vi "Set Serial Break Event.vi"() -> ()   [LabVIEW 2023]
doc: "This example illustrates how to introduce a break in the data line during serial communication. The VISA Serial Break VI is used to introduce a break in the data line. This VI can be run alongside the Detect Serial Break Event example on a separate serial port to monitor the breaks.\n\nThe serial break is a condition that holds the transmit line logic-low for longer than one data byte. Normally, if there's no data to transmit, then the transmit line idle condition is logic-high. Your application may require that you send a serial break in the transmission line. You can use this example to provide that capability to a particular device. Alternatively, you can use this example to test the Detect Serial Break Event example."
uses:
  support/Serial - Settings.ctl
  <vilib>/Instr/_visa.llb/VISA Configure Serial Port (Instr).vi
  <vilib>/Instr/_visa.llb/VISA Serial Break (Instr).vi
panel:
  in  "Serial Settings":T1={"baud rate"=9600, "data bits"=8, "parity"=enum."None", "stop bits"=10, "flow control"=0} {"flow control" items=["None"=0, "XON/XOFF"=1, "RTS/CTS"=2, "DTR/DSR"=4]; "stop bits" items=["1.0"=10, "1.5"=15, "2.0"=20]; "data bits" min=5 max=8 step=1; "baud rate" items=["75"=75, "110"=110, "134"=134, "150"=150, "300"=300, "600"=600, "1200"=1200, "1800"=1800, "2400"=2400, "4800"=4800, "7200"=7200, "9600"=9600, "14400"=14400, "19200"=19200, "28800"=28800, "38400"=38400, "56000"=56000, "57600"=57600, "115200"=115200, "128000"=128000, "230400"=230400]}
  in  "break length":i16=250 min=1 max=500
  in  "Set Break":bool
  in  "Stop":bool
  in  "VISA resource name":refnum<visa-resource-name>="COM1"
  # "Overview: Demonstrates the use of the VISA functions to set a break in the line during serial communication.\nRequirements: NI-VISA Driver, multiple serial ports\nInstructions:\n1. Ensure Detect Serial Break Event.vi is already running.\n2. Ensure that the VISA resource name values in both VIs are set to different serial ports that are connected to each other.\n3. Run the VI.\n4. Click the Set Break button and observe the front panel of Detect Serial Break Event.vi. You should see the Break Detected? light come on, and the Number of Breaks indicator increment by 1.\n5. Click Stop to stop the VI."
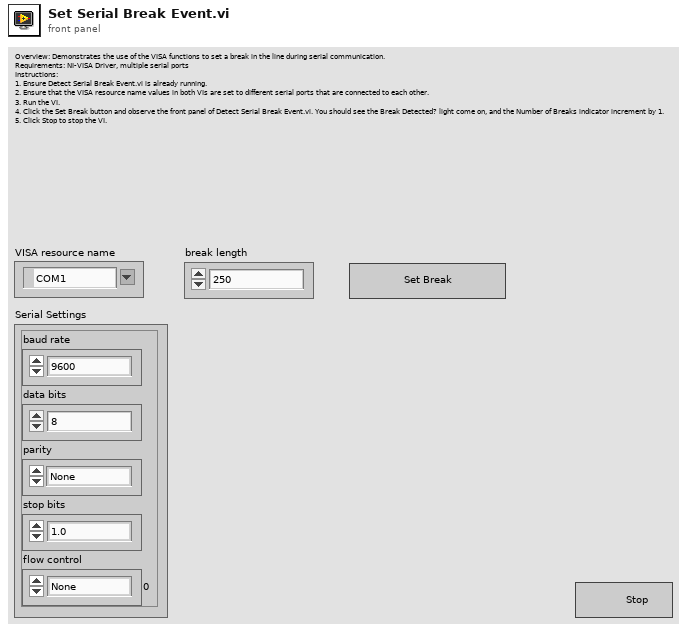
[diagram p1: front panel]
types:
  T1 = typedef "Serial - Settings.ctl" = cluster{"baud rate":u32, "data bits":u16, "parity":enum16{"None", "Odd", "Even", "Mark", "Space"}, "stop bits":u16, "flow control":u16}
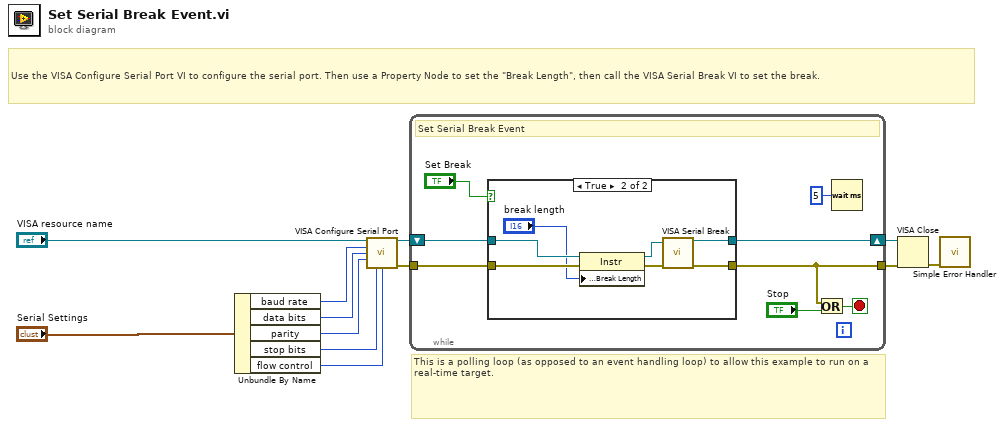
[diagram p0: block diagram]
diagram:
  # "This is a polling loop (as opposed to an event handling loop) to allow this example to run on a real-time target."
  # "Use the VISA Configure Serial Port VI to configure the serial port. Then use a Property Node to set the \"Break Length\", then call the VISA Serial Break VI to set the break."
  n1 = Unbundle By Name("Serial Settings") -> ("baud rate"=w5:u32, "data bits"=w4:u16, "parity"=w3:enum16{"None", "Odd", "Even", "Mark", "Space"}, "stop bits"=w2:u16, "flow control"=w1:u16)
  n2 = call-poly "VISA Configure Serial Port"("VISA resource name"="VISA resource name", "baud rate (9600)"=w5, "data bits (8)"=w4, "parity (0:none)"=w3, "stop bits (10: 1 bit)"=w2, "flow control (0:none)"=w1) -> ("VISA resource name out"=w11:refnum<visa-resource-name>, "error out"=w10:errorcluster)  [unwired: 3 in, 5 out]
  n3 = while {
    tunnel: w10 -> [w19]
    tunnel: [w17] -> w9
    shift-right: [w18] -> w8
    shift-left: w11 -> [w20]
    stop <- w16 stop-if-true
    # "Set Serial Break Event"
    n4 = case shown="True" "Set Break" {
      tunnel: w20 -> [w21 w29]
      tunnel: w19 -> [w22 w28]
      tunnel: [w21 w27] -> w18
      tunnel: [w22 w26] -> w17
      frame False {
      }
      frame True {
        n5 = property class="Instr"(reference=w29, error in=w28, "Serial Settings:Break Length"="break length") -> (reference out=w23:refnum<visa-resource-name>, error out=w25:errorcluster)
        n6 = call-poly <vilib>:"VISA Serial Break.vi"("error in (no error)"=w25, "VISA resource name"=w23) -> ("error out"=w26:errorcluster, "VISA resource name out"=w27:refnum<visa-resource-name>)  [unwired: 2 out]
      }
    }
    n7 = Or(x=w17, y="Stop") -> (x .or. y?=w16:bool)
    n8 = Wait (ms)(milliseconds to wait=u32 5) -> ()  [unwired: 1 out]
  }
  n9 = VISA Close(VISA resource name=w8, error in (no error)=w9) -> (error out=w7:errorcluster)
  n10 = call <vilib>:"Simple Error Handler.vi"("error in (no error)"=w7) -> ()  [unwired: 4 in, 5 out]
